vi "Untitled 2 (SubVI).vi"(0 "Signal type":T1(ring), 1 "Sine frequency":dbl(slide) scale=10.0..100.0, 2 "Samples":i32, 3 "Out":bool, 5 "?":dbl(slide) scale=100.0..1000.0, 7 "Frequency":dbl(knob) scale=0.0..10.0, 9 "Amplitude":dbl(slide) scale=0.0..10.0, 12 "Square wave duty cycle (%)":dbl, 13 "Noise":u16(ring) items=["Uniform White", "Periodic Random", "Poisson Noise "], 14 "Noise amplitude":dbl(knob) scale=0.0..3.0) -> (4 "Waveform Graph":dbl[](graph))   [LabVIEW 2012]
uses:
  <vilib>/Analysis/NI_AALPro.lvlib
  <vilib>/Analysis/NI_AALBase.lvlib
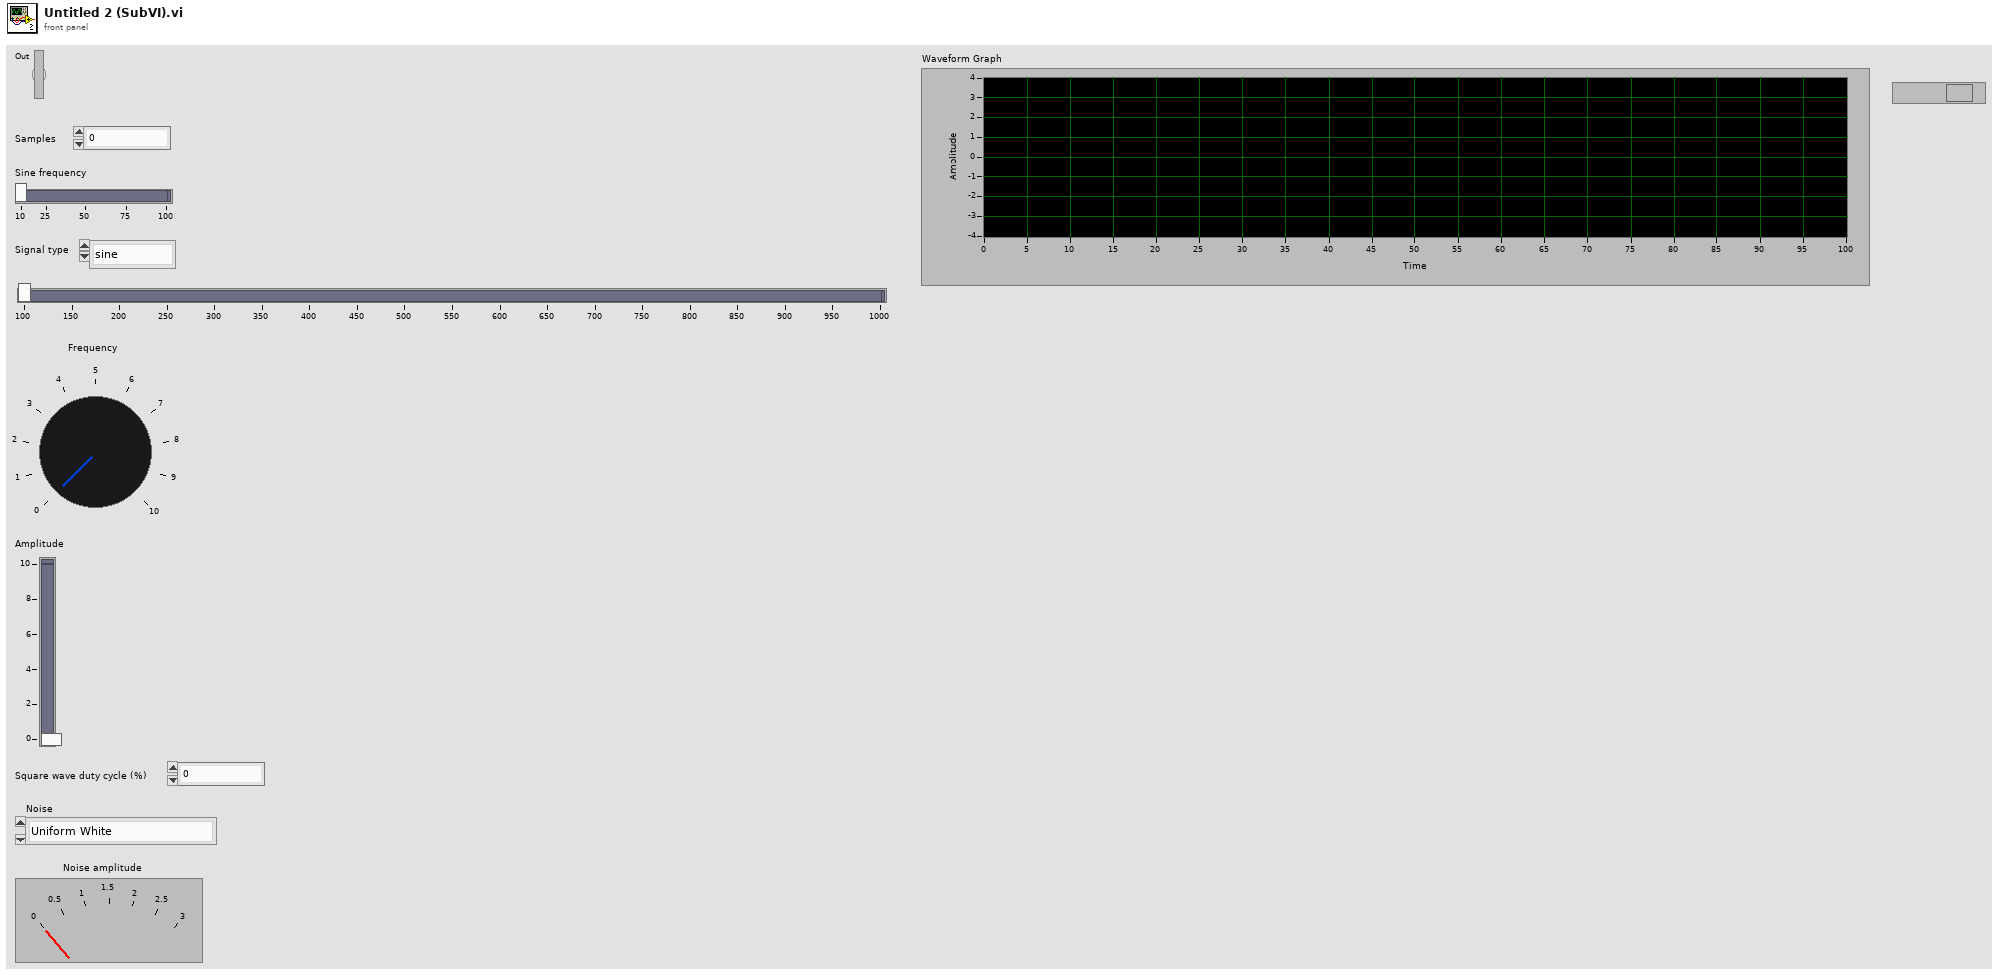
[diagram p1: front panel]
types:
  T1 = enum16{"sine", "cosine", "triangle", "square", "sawtooth", "increasing ramp", "decreasing ramp"}
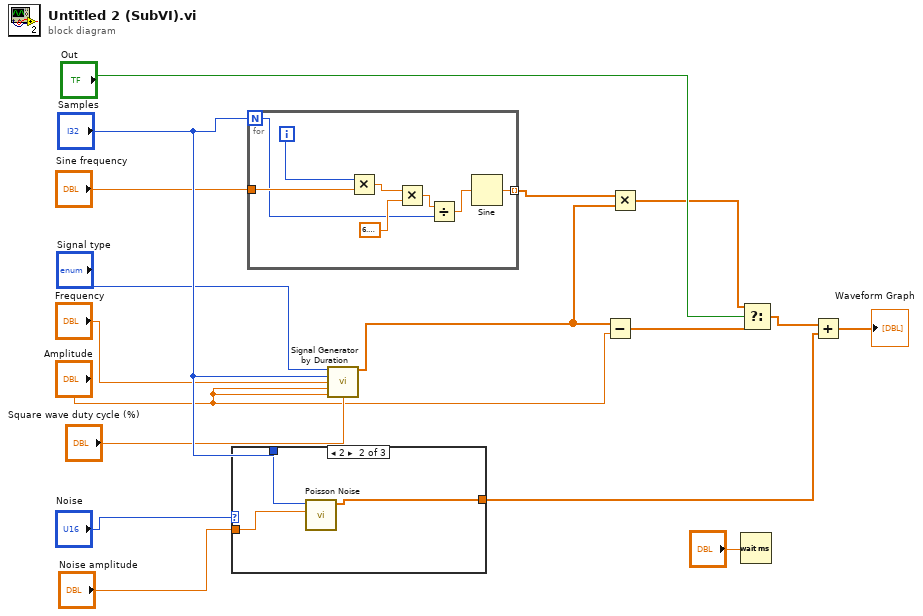
[diagram p0: block diagram]
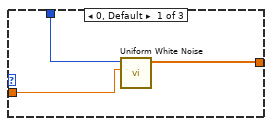
[diagram p2: hidden frame]
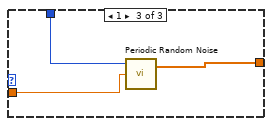
[diagram p3: hidden frame]
diagram:
  n1 = case shown="2" "Noise" {
    tunnel: "Samples" -> [w20 w23 w25]
    tunnel: "Noise amplitude" -> [w19 w22 w26]
    tunnel: [w18 w21 w24] -> w12
    frame 0, Default {
      n2 = call <vilib>:"Uniform White Noise.vi"("amplitude"=w19, "samples"=w20) -> ("uniform white noise"=w18:dbl[])  [unwired: 8 in, 1 out]
    }
    frame 2 {
      n3 = call <vilib>:"Poisson Noise.vi"("mean"=w22, "samples"=w23) -> ("poisson noise"=w21:dbl[])  [unwired: 8 in, 1 out]
    }
    frame 1 {
      n4 = call <vilib>:"Periodic Random Noise.vi"("spectral amplitude"=w26, "samples"=w25) -> ("periodic random noise"=w24:dbl[])  [unwired: 1 in, 1 out]
    }
  }
  n5 = for {
    N: "Samples" -> [w27]
    tunnel: [w32] -> w13 mode=indexing
    tunnel: "Sine frequency" -> [w34]
    i -> [w33]
    n6 = Multiply(x=w33, y=w34) -> (x*y=w31:dbl)
    n7 = Multiply(x=w31, y=6.283185307179586) -> (x*y=w29:dbl)
    n8 = Divide(x=w29, y=w27) -> (x/y=w28:dbl)
    n9 = Sine(x=w28) -> (sin(x)=w32:dbl)
  }
  n10 = call <vilib>:"Signal Generator by Duration.vi"("signal type"="Signal type", "# of samples"="Samples", "frequency"="Frequency", "amplitude"="Amplitude", "dc offset"="Amplitude", "square wave duty cycle (%)"="Square wave duty cycle (%)") -> ("signal"=w14:dbl[])  [unwired: 6 in, 3 out]
  n11 = Subtract(x=w14, y="Amplitude") -> (x-y=w3:dbl[])
  n12 = Multiply(x=w13, y=w14) -> (x*y=w2:dbl[])
  n13 = Wait (ms)(milliseconds to wait="?") -> ()  [unwired: 1 out]
  n14 = Select(t=w2, s="Out", f=w3) -> (s? t:f=w4:dbl[])
  n15 = Add(x=w4, y=w12) -> (x+y=→"Waveform Graph":dbl[])
